vi "Read delimiter.vi"(8 "error in (no error)":errorcluster, 11 "CSVLayout in":refnum<class "CSVLayout.lvclass">) -> (0 "error out":errorcluster, 2 "delimiter":string=",", 3 "CSVLayout out":refnum<class "CSVLayout.lvclass">)   [LabVIEW 2026, in "Lumberjack.lvlib" / "CSVLayout.lvclass"]
doc: "Returns the layout's single-character column delimiter.\nClass private-data accessor; reads the `delimiter` field set at layout creation, so Format needs no delimiter input. No side effects.\nLumberjack.lvlib, CSVLayout.lvclass, public."
uses:
  CSVLayout.lvclass
  CSVLayout.lvclass/CSVLayout.ctl
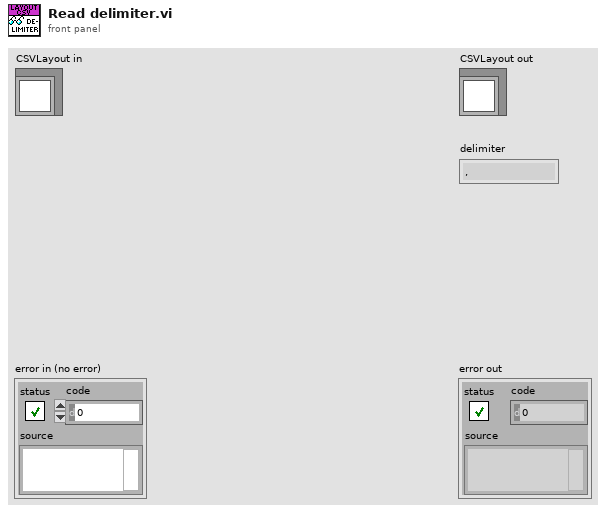
[diagram p1: front panel]
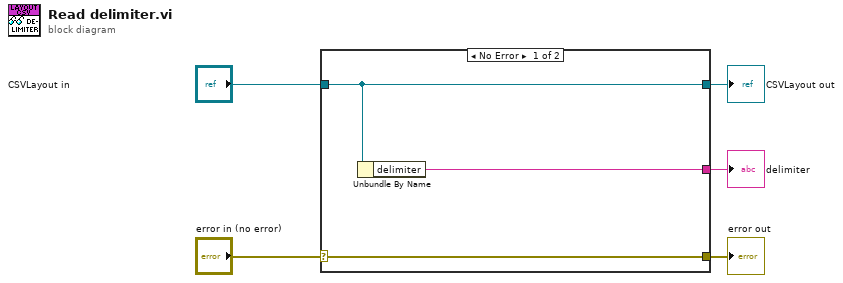
[diagram p0: block diagram]
diagram:
  n1 = case shown="No Error" "error in (no error)" {
    selector: "error in (no error)" -> [w8 w9]
    tunnel: [w8 w9] -> w4
    tunnel: [w7 w10] -> w2
    tunnel: "CSVLayout in" -> [w7 w10]
    tunnel: [w6 _] -> w1
    frame No Error {
      n2 = Unbundle By Name(w7) -> ("delimiter"=w6:string)
    }
    frame Error {
    }
  }
  "error out" <- w4
  "CSVLayout out" <- w2
  "delimiter" <- w1
